vi "GOOP_LVClass_Item_Init.vi"(11 "Object":u64) -> ()   [LabVIEW 2014]
doc: "Copyright (c) 2010 Symbio (www.symbio.com). All rights reserved."
uses:
  <resource>/Framework/Providers/Open_GDS/ClassProviders/Common/LvClass_class/GDSLvClass_IconSettingsNames.ctl
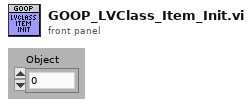
[diagram p1: front panel]
types:
  T1 = typedef "ItemRef.ctl" = u64
  T2 = typedef "GDSLvClass_IconSettingsNames.ctl" = enum16{"EndevoGOOP_ColorFrame", "EndevoGOOP_FrameThickness", "EndevoGOOP_ColorHeader", "EndevoGOOP_ColorTextHeader", "EndevoGOOP_ColorPublic", "EndevoGOOP_ColorProtected", "EndevoGOOP_ColorPrivate", "EndevoGOOP_ColorTextBody", "EndevoGOOP_ClassItemIcon", "EndevoGOOP_ClassBodyIcon"}
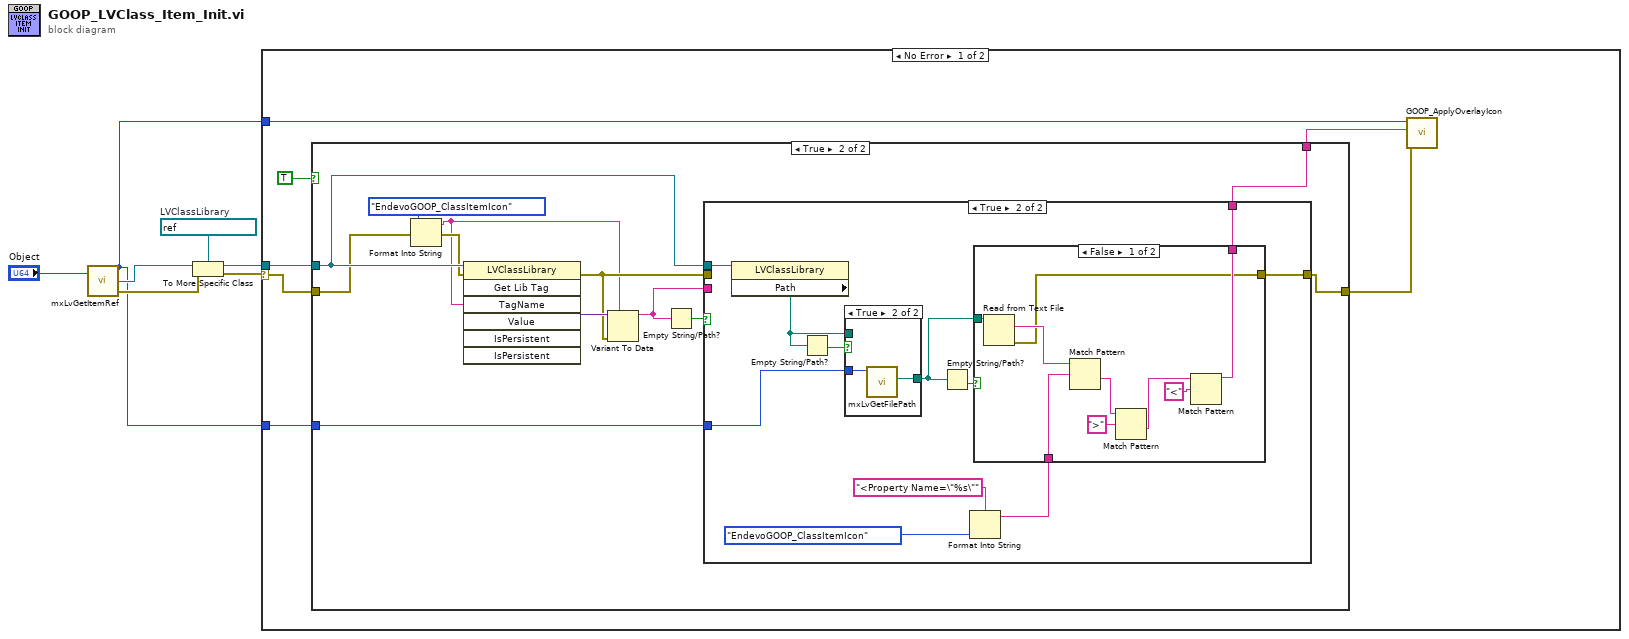
[diagram p0: block diagram]
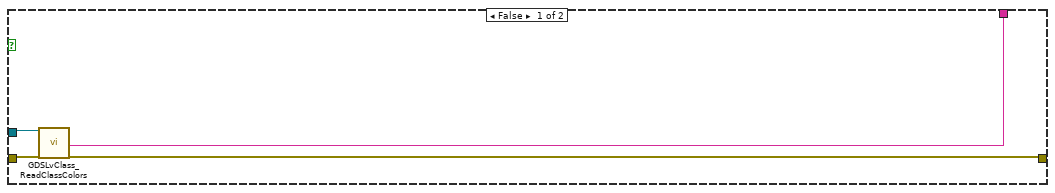
[diagram p2: hidden frame]
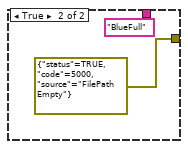
[diagram p4: hidden frame]
diagram:
  w4 = refnum<vi> refnum  # LVClassLibrary
  n1 = call <resource>:"mxLvGetItemRef.vi"("Item"="Object") -> ("Item"=w1:T1, "Item Refnum"=w6:refnum<vi>, "error out"=w3:errorcluster)  [unwired: 1 in]
  n2 = To More Specific Class(target class=w4, reference=w6, error in=w3) -> (specific class reference=w5:refnum<vi>, error out=w2:errorcluster)
  n3 = case shown="No Error" w2 {
    selector: w2 -> [w10 _]
    tunnel: w1 -> [w14 _]
    tunnel: w5 -> [w11 _]
    tunnel: w1 -> [w9 _]
    frame No Error {
      n4 = case shown="True" TRUE {
        tunnel: [w15 w30] -> w13
        tunnel: [w16 w29] -> w12
        tunnel: w11 -> [w17 w28]
        tunnel: w10 -> [w18 w27]
        tunnel: w9 -> [_ w26]
        frame False {
          n5 = call <resource>:"GDSLvClass_ReadClassColors.vi"("Library Refnum"=w17, "error in (no error)"=w18) -> ("ClassItemIconName(NoExtension)"=w16:string, "error out"=w15:errorcluster)  [unwired: 12 in, 4 out]
        }
        frame True {
          n6 = Format Into String(error in=w27, GDSLvClass_IconSettingsNames."EndevoGOOP_ClassItemIcon" ("Enum")) -> (resulting string=w20:string, error out=w23:errorcluster)  [unwired: 2 in]
          n7 = invoke class="LVClassLibrary" method="Get Lib Tag"(reference=w28, error in=w23, "TagName"=w20) -> (error out=w21:errorcluster, "Value"=w25:variant)  [unwired: 4 in, 5 out]
          n8 = Variant To Data(error in=w21, type=w20, Variant=w25) -> (data=w19:string)  [unwired: 1 out]
          n9 = Empty String/Path?(string/path=w19) -> (empty?=w22:bool)
          n10 = case shown="True" w22 {
            tunnel: w28 -> [_ w43]
            tunnel: w21 -> [w31 _]
            tunnel: [w32 w39] -> w29
            tunnel: w19 -> [w32 _]
            tunnel: [w31 w38] -> w30
            tunnel: w26 -> [_ w36]
            frame False {
            }
            frame True {
              n11 = property class="LVClassLibrary"(reference=w43) -> ("Path"=w35:path)  [unwired: 1 in, 2 out]
              n12 = Empty String/Path?(string/path=w35) -> (empty?=w37:bool)
              n13 = case shown="True" w37 {
                tunnel: w36 -> [_ w57]
                tunnel: [w55 w56] -> w34
                tunnel: w35 -> [w55 _]
                frame False {
                }
                frame True {
                  n14 = call <resource>:"mxLvGetFilePath.vi"("Item"=w57) -> ("File Path"=w56:path)  [unwired: 8 in, 2 out]
                }
              }
              n15 = Empty String/Path?(string/path=w34) -> (empty?=w33:bool)
              n16 = Format Into String(format string="<Property Name=\"%s\"", GDSLvClass_IconSettingsNames."EndevoGOOP_ClassItemIcon" ("Enum")) -> (resulting string=w40:string)  [unwired: 2 in, 1 out]
              n17 = case shown="False" w33 {
                tunnel: w40 -> [w48 _]
                tunnel: [w46 "BlueFull"] -> w39
                tunnel: [w45 errorcluster {"status"=TRUE, "code"=5000, "source"="FilePath Empty"} ("error out")] -> w38
                tunnel: w34 -> [w44 _]
                frame False {
                  n18 = Read from Text File(file (use dialog)=w44) -> (text=w47:string, error out=w45:errorcluster)  [unwired: 3 in, 2 out]
                  n19 = Match Pattern(string=w47, regular expression=w48) -> (after substring=w51:string)  [unwired: 1 in, 3 out]
                  n20 = Match Pattern(string=w51, regular expression=">") -> (after substring=w52:string)  [unwired: 1 in, 3 out]
                  n21 = Match Pattern(string=w52, regular expression="<") -> (before substring=w46:string)  [unwired: 1 in, 3 out]
                }
                frame True {
                }
              }
            }
          }
        }
      }
      n22 = call <resource>:"GOOP_ApplyOverlayIcon.vi"("error in (no error)"=w13, "IconName(NoPngExtension)"=w12, "Object"=w14) -> ()  [unwired: 8 in, 1 out]
    }
    frame Error {
    }
  }
